vi "Dashboard Main.vi"() -> ()   [LabVIEW 2019]
uses:
  <vilib>/Utility/miscctls.llb/LVRowAndColumnTypeDef.ctl
  <vilib>/event_ctls.llb/eventvkey.ctl
  <vilib>/Rock Robotics/Network Tables/NT Read Numeric Array.vi
  <vilib>/Rock Robotics/Network Tables/NT Read Boolean.vi
  <vilib>/Rock Robotics/WPI/Dashboard/WPI_DashboardLogging Global.vi
panel:
  in  "Camera Settings Right":T1={"Frame Rate"=30, "Compression"=30, "Size"=1, "DB Camera Config"=FALSE} {"Frame Rate" scale=1.0..30.0; "Compression" scale=100.0..-1.0; "Size" items=["640x480", "320x240", "160x120"]}
  in  "Camera Name Right":string(combo)="No Camera Selection"
  out "Camera Perf":string
  in  "Camera Settings":T1={"Frame Rate"=30, "Compression"=30, "Size"=1, "DB Camera Config"=FALSE} {"Frame Rate" scale=1.0..30.0; "Compression" scale=100.0..-1.0; "Size" items=["640x480", "320x240", "160x120"]}
  in  "TCP":refnum<k5>
  in  "Rec Mode":enum32{"Stop", "Record", "Playback"}(radio)
  out "Robot IP":string
  out "Image Message":string="Timeout in Camera Communications"
  in  "Dashboard Tab":T2(tab)
  in  "Select Auto":string(combo)="Select Autonomous ..."
  out "NT Connection":bool
  out "MotorChart R":cluster{"Numeric":dbl, "Numeric":dbl}(graph)
  out "MotorChart L":cluster{"Numeric":dbl, "Numeric":dbl}(graph)
  out "MotorSliders R":cluster{"MotorSlide1":dbl, "MotorSlide2":dbl} {"MotorSlide2" scale=-1.0..1.0 scale format="%#_2e"; "MotorSlide1" scale=-1.0..1.0 scale format="%#_2e"}
  out "MotorSliders L":cluster{"MotorSlide1":dbl, "MotorSlide2":dbl} {"MotorSlide2" scale=-1.0..1.0 scale format="%#_2e"; "MotorSlide1" scale=-1.0..1.0 scale format="%#_2e"}
  out "Gyro":dbl(knob) scale=0.0..360.0
  out "JS1 Z":dbl(slide) scale=-1.0..1.0 scale format="%#_2e"
  out "JS1 Graph":cluster{"X":dbl, "Y":dbl}[](graph)
  out "JS1 Buttons":T3
  out "JS2 Z":dbl(slide) scale=-1.0..1.0 scale format="%#_2e"
  out "JS2 Graph":cluster{"X":dbl, "Y":dbl}[](graph)
  out "JS2 Buttons":T3
  out "Mode":T4(ring)=enum."Auto Disabled"
  out "Right Camera Perf":cluster{"Bandwidth (Mbps)":dbl, "FPS":dbl}
  out "Camera Image Right":T5(plugin-control)
  in  "DB/String 9":string
  in  "DB/String 8":string
  in  "DB/String 7":string
  in  "DB/String 6":string
  in  "DB/String 5":string
  in  "DB/String 4":string
  in  "DB/String 3":string
  in  "DB/String 2":string
  in  "DB/String 1":string
  in  "DB/String 0":string
  in  "DB/Slider 0":dbl(slide) scale=0.0..5.0
  in  "DB/Slider 1":dbl(slide) scale=0.0..5.0
  in  "DB/Slider 2":dbl(slide) scale=0.0..5.0
  in  "DB/Slider 3":dbl(slide) scale=0.0..5.0
  out "DB/LED 3":bool
  out "DB/LED 2":bool
  out "DB/LED 1":bool
  out "DB/LED 0":bool
  in  "DB/Button 3":bool
  in  "DB/Button 2":bool
  in  "DB/Button 1":bool
  in  "DB/Button 0":bool caption="New Name"
  out "Locked On":bool
  out "Current Shot":string
  out "Has Goal Target":bool
  out "Extendo Locked":bool
  out "Collector Position":string
  out "Ball Count":i32(slide) scale=0.0..5.0
  out "Spinny Thingy Color":string
  in  "Autonomous Mode":string(combo)
  in  "Test Slider":dbl(slide) scale=0.0..100.0 scale format="%#_3g"
  in  "On/Off":bool caption="Solenoid"
  in  "Test Name":u16(ring) items=["Select the test to run..."]
  in  "Test Tree":string(tree)
  in  "Motor":cluster{"Value":dbl, "Enable":bool} {"Value" scale=-1.0..1.0 scale format="%#_3g"}
  out "Progress":T6 {"Test Progress" scale=0.0..100.0}
  in  "Rev/Fwd":cluster{"Forward":bool, "Reverse":bool}
  in  "Test Ring":u16(ring) items=["Monochrome", "Color"]
  out "Cmd Status":string
  in  "Execute Command":bool
  in  "Command Params":string[][](table)
  in  "Command Selection":i32(listbox)
  in  "CheckList":i32(listbox)
  out "Tree":string(tree)
  out "Camera Image":T5(plugin-control)
  out "Background":bool
  in  "Camera Name":string(combo)="No Camera Selection"
  # "HW"
  # "HW"
  # "Joysticks"
  # "Drive Motors"
  # "Front"
  # "Right"
  # "Left"
  # "Back"
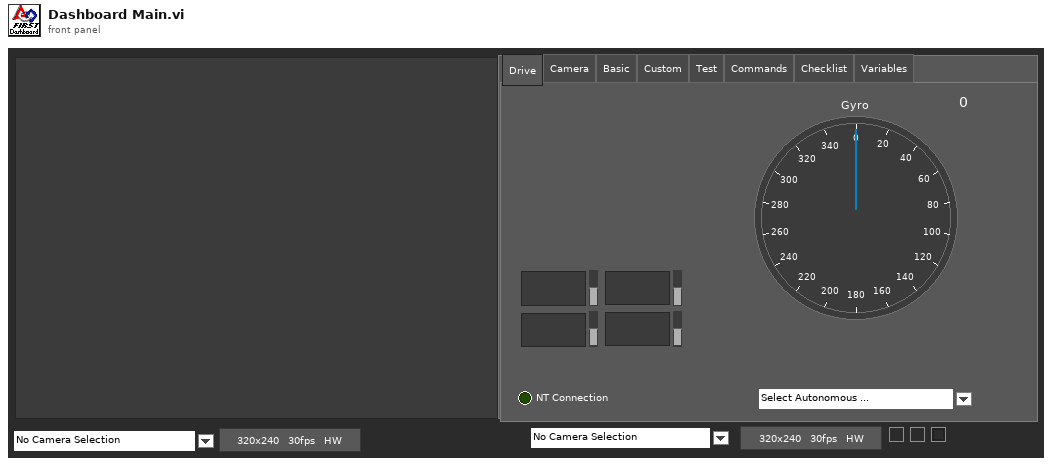
[diagram p1: front panel]
types:
  T1 = cluster{"Frame Rate":i32, "Compression":i32, "Size":u16, "DB Camera Config":bool}
  T2 = enum32{"Drive", "Camera", "Basic", "Custom", "Test", "Commands", "Checklist", "Variables"}
  T3 = cluster{bool, bool, bool, bool, bool, bool, bool, bool, bool, bool, bool, bool}
  T4 = enum8{"Tele-Op Disabled", "Tele-Op Enabled", "Auto Disabled", "Auto Enabled", "Test Disabled", "Test Enabled", "Disconnected", "No Code", "E-Stop"}
  T5 = typedef "IMAQ Image.ctl" = refnum<image>
  T6 = cluster{"Test Progress":u8, "Test Progress Text":string}
  T7 = cluster{"Save Path":path, "Interval (s)":dbl, "Keep":i32}
  T8 = typedef "Image Type" = u32
  T9 = cluster{"IDs":cluster{"RPC field ID":u16, "Unique ID":u16}, "String":string}
  T10 = cluster{"Error Strings":string, "Disable Counts":cluster{u16, u16}, "Rail Faults":cluster{u16, u16, u16}, "Robot IP":string, "DB Mode":u8, "Event Info":cluster{"Name":string, "Type":u8, "Number":u16, "Replay":u8}}
  T11 = cluster{"Storage":cluster{"Disk Free":u64, "RAM Block":u32, "RAM free":u32}, "CPU Utilization":cluster{"CPU % ISR":sgl, "CPU % Time Crit":sgl, "CPU % Timed Str":sgl, "CPU % High":sgl, "CPU % Above":sgl, "CPU % Normal":sgl, "CPU % Low":sgl}, "CAN":cluster{"% Bus Utilization":sgl, "Bus Off Cnt":u32, "TX_FIFO Full Cnt":u32, "Receive Error Cnt":u8, "Transmit Error Cnt":u8}, "HID":cluster{"HID Outputs":u32, "Rumble Low":u16, "Rumble High":u16}[]}
  T12 = cluster{"Status bits":cluster{"Test Mode":bool, "Autonomous":bool, "Enabled":bool, "Code Start":bool, "Brownout":bool, "Reserved 2":bool, "Reserved 3":bool, "E-Stop":bool}, "Code Trace":cluster{"Disabled":bool, "TeleOp":bool, "Auto":bool, "Test":bool}, "Controller Type":enum16{"unknown", "cRIO", "roboRio"}, "Code?":enum16{"unknown", "noCode", "code"}, "Battery V":dbl}
  T13 = cluster{"Control Bits":cluster{"TestMode":bool, "Autonomous":bool, "Enabled":bool, "FMS Present":bool, bool, bool, bool, "E-Stop":bool}, "Team Station ":u8, "Countdown":sgl, "Joystick Values":cluster{"Axes":dbl[], "Buttons":bool[], "POVs":i16[]}[]}
  T14 = cluster{"Axes":dbl[], "Buttons":bool[], "POVs":i16[]}[]
  T15 = cluster{"Axes":dbl[], "Buttons":bool[], "POVs":i16[]}
  T16 = cluster{"Buttons[0]":bool, "Buttons[1]":bool, "Buttons[2]":bool, "Buttons[3]":bool, "Buttons[4]":bool, "Buttons[5]":bool, "Buttons[6]":bool, "Buttons[7]":bool, "Buttons[8]":bool, "Buttons[9]":bool, "Buttons[10]":bool, "Buttons[11]":bool}
  T17 = cluster{"Camera Image":refnum<vi>, "Dashboard Tab":refnum<vi>, "Background":refnum<vi>, "Rec Mode":refnum<vi>, "Test Slider":refnum<vi>, "On/Off ":refnum<vi>, "Test Ring":refnum<vi>, "Rev/Fwd":refnum<vi>, "Test Name":refnum<vi>, "Motor":refnum<vi>, "Progress":refnum<vi>, "CheckList":refnum<vi>, "Tree":refnum<vi>, "Test Tree":refnum<vi>, "Command Params":refnum<vi>, "Command Selection":refnum<vi>, "Execute Command":refnum<vi>, "Cmd Status":refnum<vi>, "Camera Settings":refnum<vi>, "Camera Name":refnum<vi>, "Camera Perf":refnum<vi>, "Camera Settings Right":refnum<vi>, "Camera Name Right":refnum<vi>, "Camera Image Right":refnum<vi>}
  T18 = cluster{"Global Rectangle":i32[], "Contours":cluster{"Contour Type":u32, "ROI Type":u32, "Points":i32[]}[]}
  T19 = cluster{"Camera Name":string, string, "Saved DB Images Info":cluster{"Save Path":path, "Interval (s)":dbl, "Keep":i32}}
  T20 = cluster{"Camera Name Right":string, string, "Saved DB Images Info":cluster{"Save Path":path, "Interval (s)":dbl, "Keep":i32}}
  T21 = cluster{"Operation":enum16{"Update", "Clear"}, "Color Box":u32}[]
  T22 = typedef "eventvkey.ctl" = enum16{"ASCII", "Enter", "Return", "Shift", "Ctrl", "Alt", "Cmd", "Opt", "Caps", "NumLock", "Clear", "Break", "Up", "Down", "Left", "Right", "Insert", "Delete", "Home", "End", "PageUp", "PageDown", "Escape", "Help", "Pause", "ScrollLock", "F1", "F2", "F3", "F4", "F5", "F6", "F7", "F8", "F9", "F10", "F11", "F12", "F13", "F14", "F15", "F16", "F17", "F18", "F19", "F20", "F21", "F22", "F23", "F24", "Play", "VolumeUp", "VolumeDown", "Mute", "Two Byte Char"}
  T23 = cluster{"Image Size":bool, "Image Type":bool, "Pixel Value":bool, "ROI Information":bool, "Zoom Factor":bool}
  T24 = cluster{"Operation":enum16{"Update", "Clear"}, "Color Box":u32}
  T25 = typedef "LVRowAndColumnTypeDef.ctl" = cluster{"Row":i32, "Column":i32}
  T26 = cluster{"Shift":bool, "Ctrl":bool, "Alt":bool, "Cmd":bool, "Opt":bool}
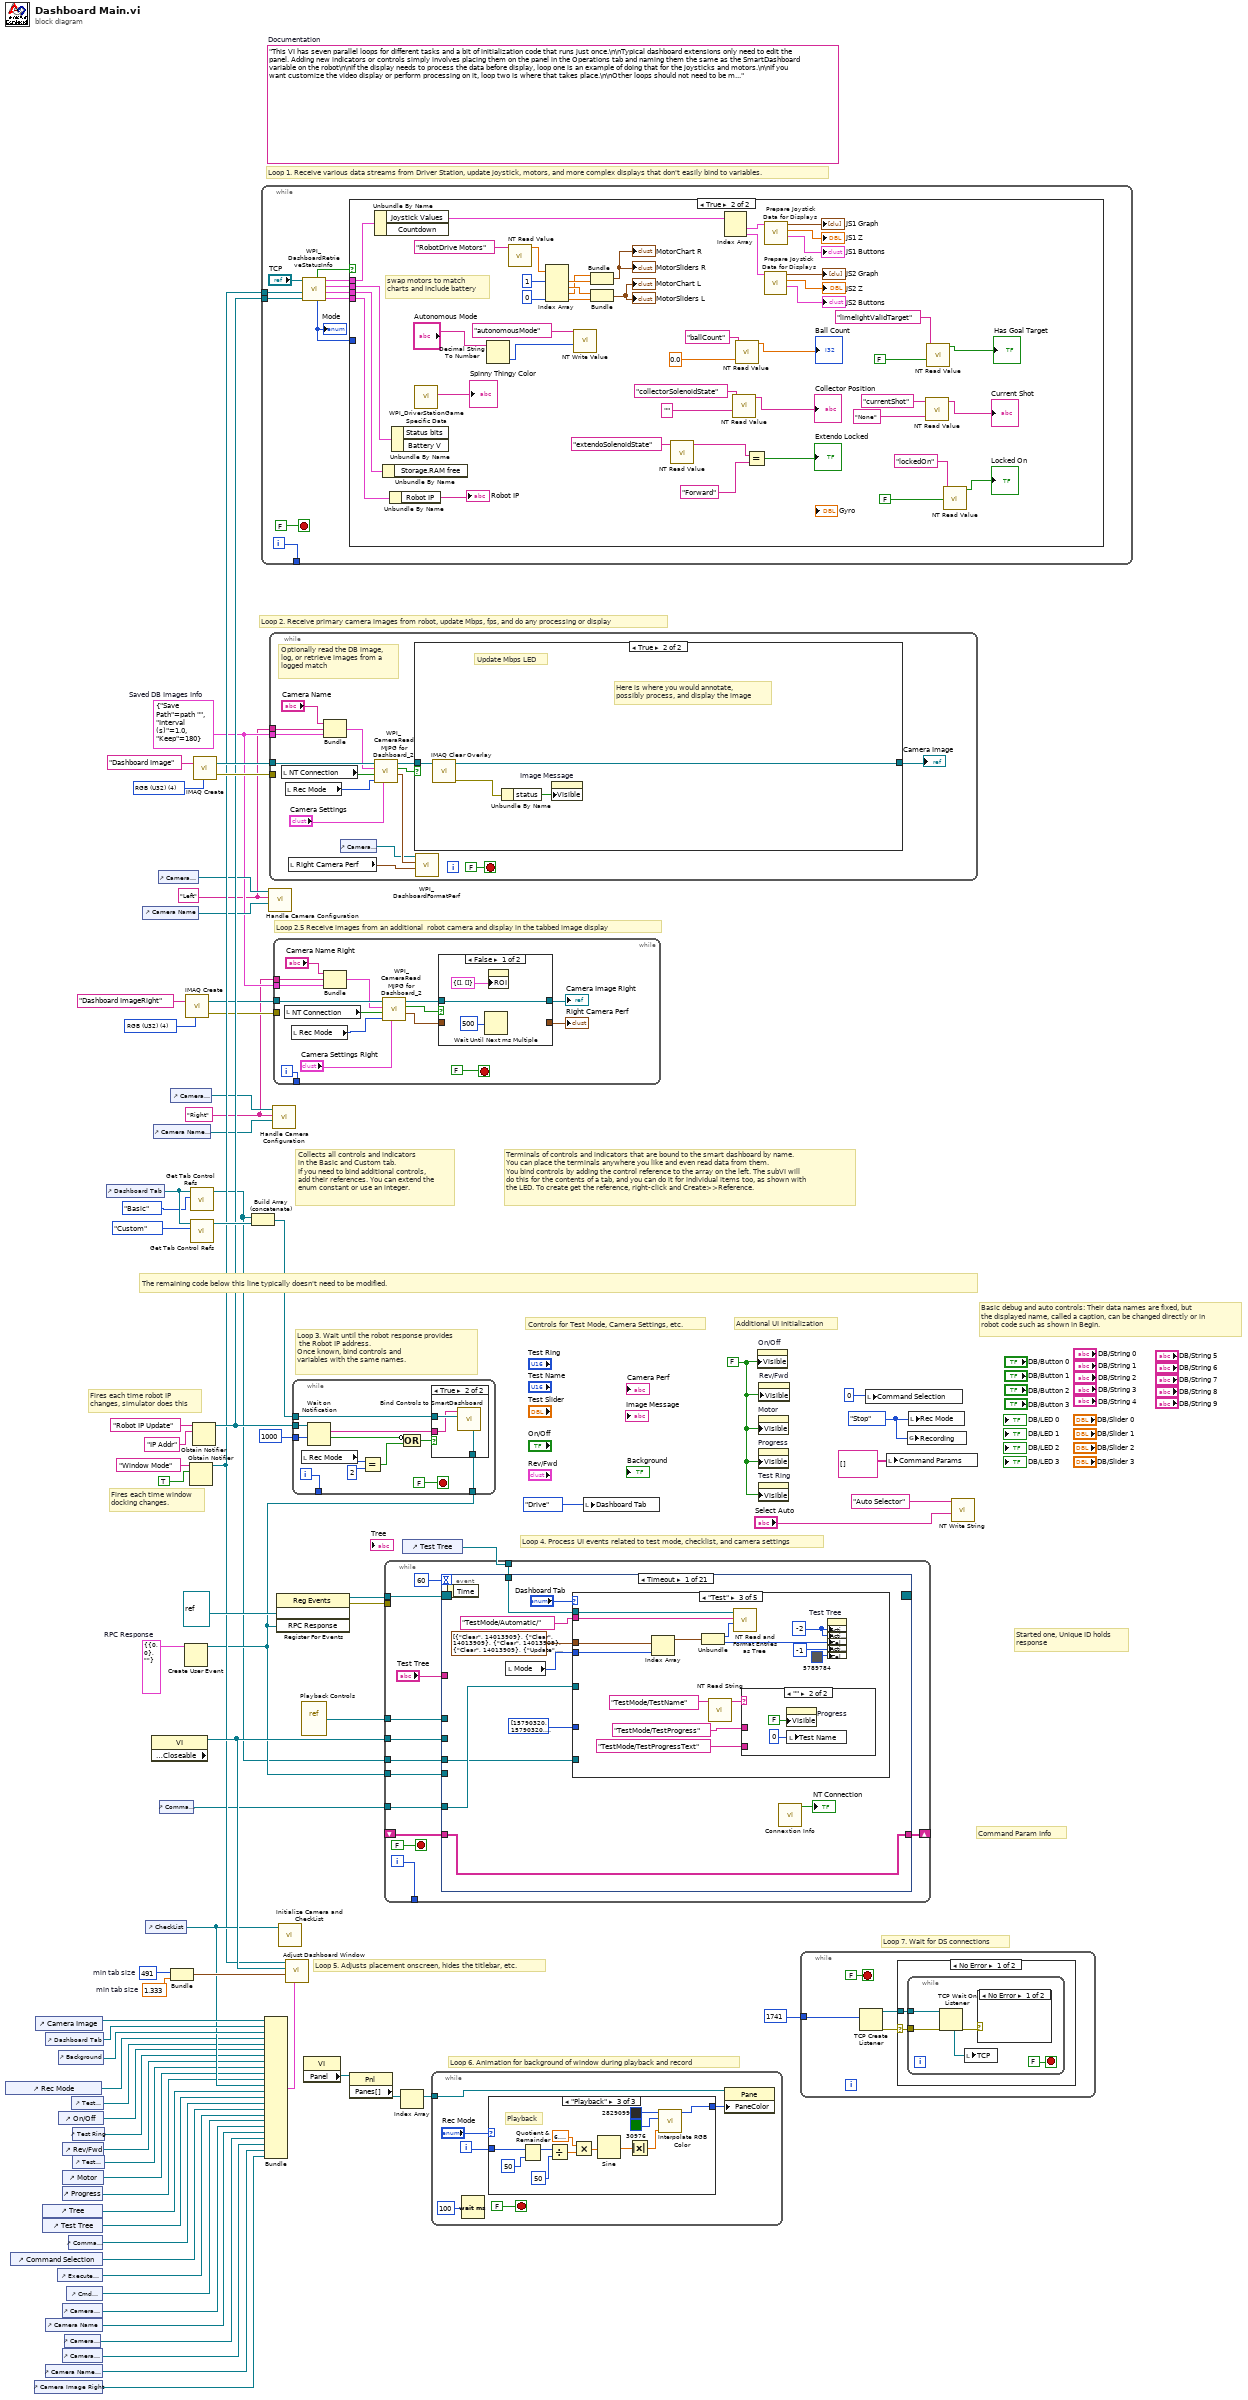
[diagram p0: block diagram]
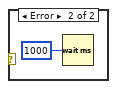
[diagram p3: hidden frame]
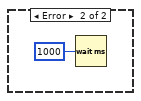
[diagram p4: hidden frame]
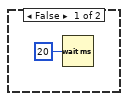
[diagram p5: hidden frame]
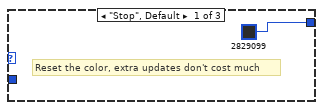
[diagram p6: hidden frame]
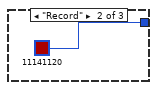
[diagram p7: hidden frame]
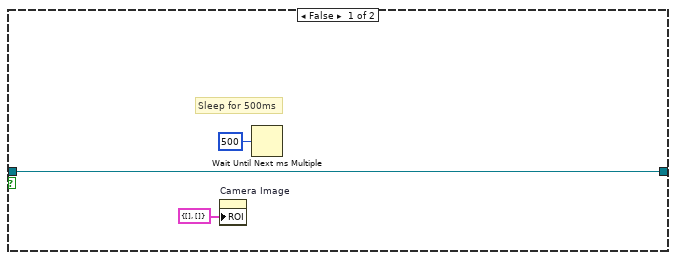
[diagram p9: hidden frame]
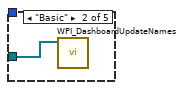
[diagram p11: hidden frame]
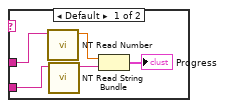
[diagram p12: hidden frame]
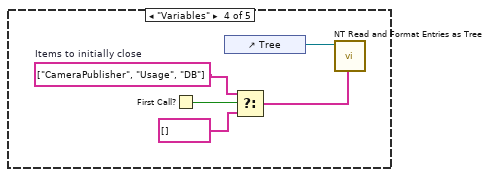
[diagram p13: hidden frame]
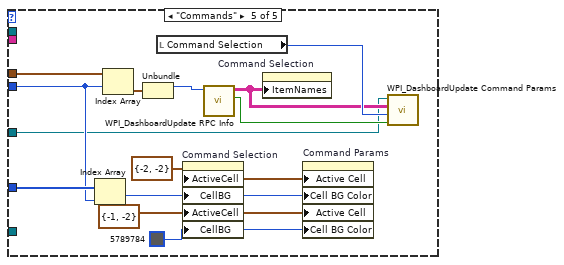
[diagram p14: hidden frame]
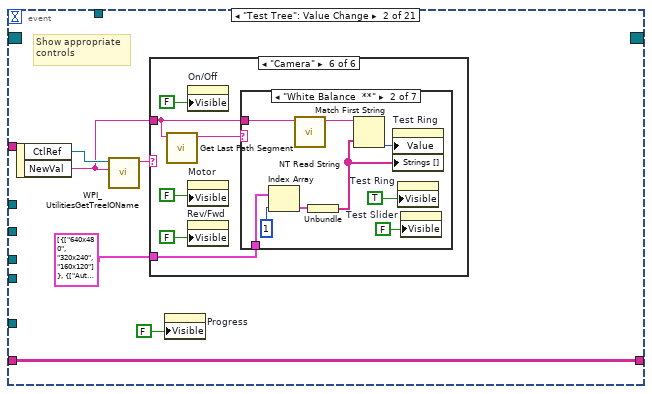
[diagram p15: hidden frame]
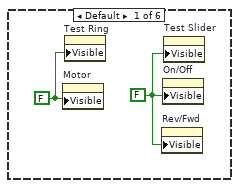
[diagram p16: hidden frame]
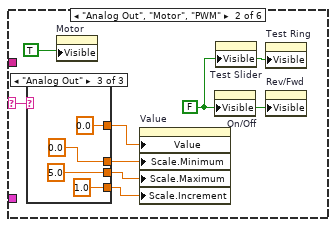
[diagram p17: hidden frame]
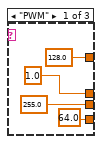
[diagram p18: hidden frame]
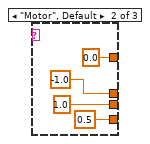
[diagram p19: hidden frame]
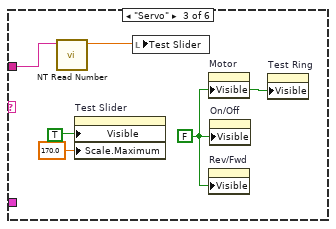
[diagram p20: hidden frame]
diagram:
  w3 = T7 {"Save Path"=path "", "Interval (s)"=1.0, "Keep"=180}  # Saved DB Images Info
  w2 = "Right"
  w1 = "Left"
  w13 = T8 4 items=["Grayscale (U8)", "Grayscale (I16)", "Grayscale (SGL)", "Complex (CSG)", "RGB (U32)", "HSL (U32)", "RGB (U64)"] ("Image Type")
  w29 = T9 {"IDs"={"RPC field ID"=0, "Unique ID"=0}, "String"=""}  # RPC Response
  w52 = 491  # min tab size
  w51 = 1.333  # min tab size
  w59 = enum32{"Stop", "Record", "Playback"}."Stop" ("Rec Mode")
  w36 = FALSE ("Visible")
  (unwired) "This VI has seven parallel loops for different tasks and a bit of initialization code that runs just once.\n\nTypical dashboard extensions only need to edit the panel. Adding new indicators or controls simply involves placing them on the panel in the Operations tab and naming them the same as the SmartDashboard variable on the robot\n\nIf the display needs to process the data before display, loop one is an example of doing that for the joysticks and motors.\n\nIf you want customize the video display or perform processing on it, loop two is where that takes place.\n\nOther loops should not need to be modified. They are pretty standard, and document the task they perform."  # Documentation
  w76 = T8 4 items=["Grayscale (U8)", "Grayscale (I16)", "Grayscale (SGL)", "Complex (CSG)", "RGB (U32)", "HSL (U32)", "RGB (U64)"] ("Image Type")
  # "Loop 2.5 Receive images from an additional  robot camera and display in the tabbed image display"
  # "Command Param Info"
  # "Started one, Unique ID holds\nresponse"
  # "Loop 7. Wait for DS connections"
  # "Basic debug and auto controls: Their data names are fixed, but\nthe displayed name, called a caption, can be changed directly or in\nrobot code such as shown in Begin."
  # "Controls for Test Mode, Camera Settings, etc."
  # "Additional UI Initialization"
  # "Loop 6. Animation for background of window during playback and record"
  # "Fires each time robot IP\nchanges, simulator does this"
  # "Fires each time window\ndocking changes."
  # "Collects all controls and indicators\nin the Basic and Custom tab.\nIf you need to bind additional controls,\nadd their references. You can extend the\nenum constant or use an integer."
  # "The remaining code below this line typically doesn't need to be modified."
  # "Loop 4. Process UI events related to test mode, checklist, and camera settings"
  # "Terminals of controls and indicators that are bound to the smart dashboard by name.\nYou can place the terminals anywhere you like and even read data from them.\nYou bind controls by adding the control reference to the array on the left. The subVI will\ndo this for the contents of a tab, and you can do it for individual items too, as shown with\nthe LED. To create get the reference, right-click and Create>>Reference."
  # "Loop 3. Wait until the robot response provides\n the Robot IP address.\nOnce known, bind controls and\nvariables with the same names."
  # "Loop 5. Adjusts placement onscreen, hides the titlebar, etc."
  # "Loop 1. Receive various data streams from Driver Station, update joystick, motors, and more complex displays that don't easily bind to variables."
  # "Loop 2. Receive primary camera images from robot, update Mbps, fps, and do any processing or display"
  n1 = control-ref of="Rec Mode"() -> (w42:refnum<vi>)
  n2 = control-ref of="Command Selection"() -> (w28:refnum<vi>)
  n3 = control-ref of="Camera Image Right"() -> (w6:refnum<vi>)
  n4 = control-ref of="Camera Image"() -> (w54:refnum<vi>)
  n5 = control-ref of="Tree"() -> (w46:refnum<vi>)
  n6 = control-ref of="Test Tree"() -> (w45:refnum<vi>)
  n7 = control-ref of="Dashboard Tab"() -> (w53:refnum<vi>)
  n8 = control-ref of="Camera Name"() -> (w19:refnum<vi>)
  n9 = control-ref of="Camera Name Right"() -> (w7:refnum<vi>)
  n10 = control-ref of="Execute Command"() -> (w30:refnum<vi>)
  n11 = control-ref of="Background"() -> (w49:refnum<vi>)
  n12 = control-ref of="On/Off"() -> (w40:refnum<vi>)
  n13 = control-ref of="Progress"() -> (w37:refnum<vi>)
  n14 = control-ref of="Camera Settings"() -> (w20:refnum<vi>)
  n15 = control-ref of="Camera Settings Right"() -> (w8:refnum<vi>)
  n16 = control-ref of="Rev/Fwd"() -> (w38:refnum<vi>)
  n17 = control-ref of="Motor"() -> (w43:refnum<vi>)
  n18 = control-ref of="Camera Perf"() -> (w18:refnum<vi>)
  n19 = control-ref of="Cmd Status"() -> (w24:refnum<vi>)
  n20 = control-ref of="Command Params"() -> (w31:refnum<vi>)
  n21 = control-ref of="Test Slider"() -> (w41:refnum<vi>)
  n22 = control-ref of="Test Ring"() -> (w39:refnum<vi>)
  n23 = control-ref of="Test Name"() -> (w44:refnum<vi>)
  n24 = control-ref of="Dashboard Tab"() -> (w57:refnum<vi>)
  n25 = control-ref of="Camera Name"() -> (w21:refnum<vi>)
  n26 = control-ref of="CheckList"() -> (w47:refnum<vi>)
  n27 = property class="VI" props=["Front Panel.Closeable"]() -> (reference out=w58:refnum<vi>)  [unwired: 2 in, 2 out]
  n28 = control-ref of="Camera Name Right"() -> (w9:refnum<vi>)
  n29 = control-ref of="Camera Settings"() -> (w22:refnum<vi>)
  n30 = control-ref of="Command Params"() -> (w23:refnum<vi>)
  n31 = control-ref of="Camera Settings Right"() -> (w10:refnum<vi>)
  n32 = Bundle("min tab size"=w52, "min tab size"=w51) -> (w50:cluster{"min tab size":i32, "min tab size":dbl})  [unwired: 1 in]
  n33 = Create User Event(user event datatype=w29) -> (user event=w25:refnum<user-event>)  [unwired: 1 in, 1 out]
  n34 = call "IMAQ Create"("Image Name"="Dashboard ImageRight", "Image Type"=w13) -> ("New Image"=w12:T5, "error out"=w11:errorcluster)  [unwired: 2 in, 1 out]
  n35 = Obtain Notifier(name (unnamed)="Window Mode", notification data type=TRUE) -> (notifier out=w34:refnum<notifier>)  [unwired: 2 in, 2 out]
  n36 = call <vilib>:"Get Tab Control Refs.vi"("Page Index"=T2."Basic" ("Dashboard Tab"), "TabControl in"=w57) -> ("ControlsOnPage"=w17:refnum<vi>[])  [unwired: 9 in]
  n37 = call <vilib>:"Get Tab Control Refs.vi"("Page Index"=T2."Custom" ("Dashboard Tab"), "TabControl in"=w57) -> ("ControlsOnPage"=w56:refnum<vi>[])  [unwired: 9 in]
  n38 = Obtain Notifier(name (unnamed)="Robot IP Update", notification data type="IP Addr" ("name (unnamed)")) -> (notifier out=w35:refnum<notifier>)  [unwired: 2 in, 2 out]
  n39 = call "IMAQ Create"("Image Name"="Dashboard Image", "Image Type"=w76) -> ("New Image"=w74:T5, "error out"=w73:errorcluster)  [unwired: 2 in, 1 out]
  n40 = Build Array (concatenate)(w17, w56) -> (w55:refnum<vi>[])
  n41 = while {
    tunnel: [w86] -> _
    tunnel: w35 -> [w80]
    tunnel: w34 -> [w77]
    i -> [w86]
    stop <- FALSE stop-if-true
    n42 = call <vilib>:"WPI_DashboardRetrieveStatusInfo.vi"("Binding Refnum"=w80, "Window Mode Notifier"=w77, "TCP Cnx"="TCP") -> ("Power and Errors"=w81:T10, "Robot Metrics"=w84:T11, "Status Info"=w85:T12, "Control Info"=w82:T13, "Robot Mode"=w79:T4, "Process?"=w83:bool)  [unwired: 3 in]
    "Mode" <- w79
    n43 = case shown="True" w83 {
      tunnel: w85 -> [_ w135]
      tunnel: w84 -> [_ w134]
      tunnel: w82 -> [_ w133]
      tunnel: w81 -> [_ w132]
      tunnel: w79 -> [_ _]
      frame False {
        n44 = Wait (ms)(milliseconds to wait=u32 20) -> ()  [unwired: 1 out]
      }
      frame True {
        # "swap motors to match\ncharts and include battery"
        n45 = Unbundle By Name(w133) -> ("Joystick Values"=w123:T14)  [unwired: 1 out]
        n46 = Unbundle By Name(w134) -> ()  [unwired: 1 out]
        n47 = Unbundle By Name(w132) -> ("Robot IP"=→"Robot IP":string)
        n48 = Unbundle By Name(w135) -> ()  [unwired: 2 out]
        n49 = call <vilib>:"WPI_DriverStationGame Specific Data.vi"() -> ("Game Specific Data"=→"Spinny Thingy Color":string)  [unwired: 11 in]
        n50 = Decimal String To Number(string="Autonomous Mode") -> (number=w110:i32)  [unwired: 2 in, 1 out]
        n51 = call-poly <vilib>:"NT Read Value.vi"("Name"="RobotDrive Motors") -> ("Numeric Array"=w113:dbl[])  [unwired: 9 in, 1 out]
        n52 = Index Array(array=w113, index #1=1, index #4=0) -> (element #1=w127:dbl, element #2=w128:dbl, element #3=w126:dbl, element #4=w131:dbl)  [unwired: 2 in]
        n53 = call-poly <vilib>:"NT Write Value.vi"("Numeric"=w110, "Name"="autonomousMode") -> ()  [unwired: 9 in, 1 out]
        n54 = Bundle("Numeric"=w126, "Numeric"=w127) -> (→"MotorChart R" →"MotorSliders R":cluster{"Numeric":dbl, "Numeric":dbl})  [unwired: 1 in]
        n55 = Bundle("Numeric"=w128, "Numeric"=w131) -> (→"MotorChart L" →"MotorSliders L":cluster{"Numeric":dbl, "Numeric":dbl})  [unwired: 1 in]
        n56 = call-poly <vilib>:"NT Read Value.vi"("Name"="extendoSolenoidState") -> ("String"=w100:string)  [unwired: 9 in, 1 out]
        n57 = Index Array(array=w123) -> (element #1=w122:T15, element #2=w118:T15)  [unwired: 2 in]
        n58 = call-poly <vilib>:"NT Read Value.vi"("Default Value"="", "Name"="collectorSolenoidState") -> ("String"=→"Collector Position":string)  [unwired: 8 in, 1 out]
        n59 = call-poly <vilib>:"NT Read Value.vi"("Default Value"=0.0, "Name"="ballCount") -> ("Numeric"=→"Ball Count":dbl)  [unwired: 8 in, 1 out]
        n60 = Equal?(x=w100, y="Forward") -> (x = y?=→"Extendo Locked":bool)
        n61 = call "Prepare Joystick Data for Displays.vi"("Joystick Values"=w118) -> ("Buttons"=→"JS2 Buttons":T16, "Z Axis"=→"JS2 Z":dbl, "Cartesian Data"=→"JS2 Graph":cluster{"X axis":dbl, "X axis":dbl}[])  [unwired: 8 in]
        n62 = call "Prepare Joystick Data for Displays.vi"("Joystick Values"=w122) -> ("Buttons"=→"JS1 Buttons":T16, "Z Axis"=→"JS1 Z":dbl, "Cartesian Data"=→"JS1 Graph":cluster{"X axis":dbl, "X axis":dbl}[])  [unwired: 8 in]
        n63 = call-poly <vilib>:"NT Read Value.vi"("Default Value"="None", "Name"="currentShot") -> ("String"=→"Current Shot":string)  [unwired: 8 in, 1 out]
        n64 = call-poly <vilib>:"NT Read Value.vi"("Default Value"=FALSE, "Name"="limelightValidTarget") -> ("Boolean"=→"Has Goal Target":bool)  [unwired: 8 in, 1 out]
        n65 = call-poly <vilib>:"NT Read Value.vi"("Default Value"=FALSE, "Name"="lockedOn") -> ("Boolean"=→"Locked On":bool)  [unwired: 8 in, 1 out]
      }
    }
  }
  n66 = Bundle("Camera Image"=w54, "Dashboard Tab"=w53, "Background"=w49, "Rec Mode"=w42, "Test Slider"=w41, "On/Off"=w40, "Test Ring"=w39, "Rev/Fwd"=w38, "Test Name"=w44, "Motor"=w43, "Progress"=w37, "CheckList"=w47, "Tree"=w46, "Test Tree"=w45, "Command Params"=w31, "Command Selection"=w28, "Execute Command"=w30, "Cmd Status"=w24, "Camera Settings"=w20, "Camera Name"=w19, "Camera Perf"=w18, "Camera Settings Right"=w8, "Camera Name Right"=w7, "Camera Image Right"=w6) -> (w48:T17)  [unwired: 1 in]
  n67 = call "Handle Camera Configuration.vi"("CameraNameRef"=w21, "Display Name"=w1, "ClusterRef"=w22) -> ()  [unwired: 9 in]
  n68 = while {
    tunnel: w74 -> [w149]
    tunnel: w73 -> [_]
    tunnel: w3 -> [w142]
    tunnel: w1 -> [w139]
    stop <- FALSE stop-if-true
    # "Optionally read the DB image,\nlog, or retrieve images from a\nlogged match"
    n69 = local read "NT Connection"() -> (w143:bool)
    n70 = local read "Rec Mode"() -> (w146:enum32{"Stop", "Record", "Playback"})
    n71 = local read "Right Camera Perf"() -> (w137:cluster{"Bandwidth (Mbps)":dbl, "FPS":dbl})
    n72 = Bundle("Camera Name"="Camera Name", w139, "Saved DB Images Info"=w142) -> (w141:T19)  [unwired: 1 in]
    n73 = control-ref of="Camera Perf"() -> (w136:refnum<vi>)
    n74 = call <vilib>:"WPI_CameraRead MJPG for Dashboard_2.vi"("Camera Settings"="Camera Settings", "Rec Mode"=w146, "NT Connection"=w143, "Capture Info"=w141, "Image in"=w149) -> ("perf info"=w138:cluster{"Bandwidth (Mbps)":dbl, "fps":dbl}, "Active"=w147:bool, "Image\\ out"=w148:T5)  [unwired: 4 in]
    n75 = case shown="True" w147 {
      tunnel: w148 -> [w152 w155]
      tunnel: [w152 w154] -> w144
      frame False {
        # "Sleep for 500ms"
        n76 = property on="Camera Image" class="ImageControl"("ROI"=T18 {"Global Rectangle"=[], "Contours"=[]}) -> ()  [unwired: 2 in, 2 out]
        n77 = Wait Until Next ms Multiple(millisecond multiple=u32 500) -> ()  [unwired: 1 out]
      }
      frame True {
        # "Here is where you would annotate,\npossibly process, and display the image"
        # "Update Mbps LED"
        n78 = call "IMAQ Clear Overlay"("Image"=w155) -> ("error out"=w156:errorcluster, "Image Out"=w154:T5)  [unwired: 2 in, 7 out]
        n79 = Unbundle By Name(w156) -> ("status"=w157:bool)
        n80 = property on="Image Message" class="Str"("Visible"=w157) -> ()  [unwired: 2 in, 2 out]
      }
    }
    "Camera Image" <- w144
    n81 = call <vilib>:"WPI_DashboardFormatPerf.vi"("Right Camera Perf"=w137, "Performance"=w138, "String in"=w136) -> ()  [unwired: 9 in]
  }
  n82 = call "Handle Camera Configuration.vi"("CameraNameRef"=w9, "Display Name"=w2, "ClusterRef"=w10) -> ()  [unwired: 9 in]
  n83 = while {
    tunnel: w12 -> [w172]
    tunnel: w11 -> [_]
    tunnel: [w167] -> _
    tunnel: w3 -> [w163]
    tunnel: w2 -> [w160]
    i -> [w167]
    stop <- FALSE stop-if-true
    n84 = local read "NT Connection"() -> (w164:bool)
    n85 = local read "Rec Mode"() -> (w171:enum32{"Stop", "Record", "Playback"})
    n86 = Bundle("Camera Name Right"="Camera Name Right", w160, "Saved DB Images Info"=w163) -> (w162:T20)  [unwired: 1 in]
    n87 = call <vilib>:"WPI_CameraRead MJPG for Dashboard_2.vi"("Camera Settings"="Camera Settings Right", "Rec Mode"=w171, "NT Connection"=w164, "Capture Info"=w162, "Image in"=w172) -> ("perf info"=w158:cluster{"Bandwidth (Mbps)":dbl, "fps":dbl}, "Active"=w166:bool, "Image\\ out"=w169:T5)  [unwired: 4 in]
    n88 = case shown="False" w166 {
      tunnel: w169 -> [w174 w177]
      tunnel: [w174 w177] -> w165
      tunnel: [_ w176] -> w159
      tunnel: w158 -> [_ w176]
      frame False {
        n89 = Wait Until Next ms Multiple(millisecond multiple=u32 500) -> ()  [unwired: 1 out]
        n90 = property on="Camera Image Right" class="ImageControl"("ROI"=T18 {"Global Rectangle"=[], "Contours"=[]}) -> ()  [unwired: 2 in, 2 out]
      }
      frame True {
      }
    }
    "Camera Image Right" <- w165
    "Right Camera Perf" <- w159
  }
  n91 = register-events(refnum<vi> refnum, w25) -> (reference out=w63:refnum<event-registration>, error out=w62:errorcluster)  [unwired: 2 in]
  n92 = call "Initialize Camera and CheckList.vi"("ListBox in"=w47) -> ()  [unwired: 11 in]
  n93 = call "Adjust Dashboard Window.vi"("Sizing Refnums"=w48, "Size Constraints"=w50, "VI"=w58, "WIn Mode"=w34) -> ()  [unwired: 8 in]
  n94 = while {
    tunnel: w55 -> [w189]
    tunnel: w35 -> [w187]
    tunnel: [w185] -> _
    tunnel: u32 1000 ("milliseconds to wait") -> [w184]
    tunnel: w25 -> [w178]
    i -> [w185]
    stop <- FALSE stop-if-true
    n95 = local read "Rec Mode"() -> (w180:enum32{"Stop", "Record", "Playback"})
    n96 = Wait on Notification(notifier=w187, timeout in ms (-1)=w184) -> (notification=w186:string, timed out?=w182:bool)  [unwired: 2 in, 2 out]
    n97 = Equal?(x=w180, y=u16 2 ("Rec Mode")) -> (x = y?=w181:bool)
    n98 = Compound Arithmetic op=OR(invert w182, w181) -> (w183:bool)
    n99 = case shown="True" w183 {
      tunnel: w189 -> [_ w192]
      tunnel: w186 -> [_ w191]
      tunnel: w178 -> [_ w190]
      frame False {
      }
      frame True {
        n100 = call <vilib>:"Bind Controls to SmartDashboard.vi"("RPC ref"=w190, "Bound Control Refs"=w192, "Server IP Address"=w191) -> ()  [unwired: 9 in]
      }
    }
  }
  n101 = vi-ref "Playback Controls.vi"() -> (w64:refnum<vi>)
  n102 = property class="VI"() -> ("Panel"=w66:refnum<vi>)  [unwired: 2 in, 2 out]
  n103 = property class="Pnl"(reference=w66) -> ("Panes[]"=w67:refnum<vi>[])  [unwired: 1 in, 2 out]
  n104 = Index Array(array=w67) -> (element=w65:refnum<vi>)  [unwired: 1 in]
  n105 = control-ref of="Test Tree"() -> (w68:refnum<vi>)
  n106 = while {
    tunnel: [w202] -> _
    tunnel: w68 -> [w201]
    tunnel: w64 -> [w200]
    tunnel: w63 -> [w199]
    tunnel: w62 -> [_]
    tunnel: w58 -> [w198]
    tunnel: w25 -> [w197]
    tunnel: w23 -> [w196]
    shift-right: [w195] -> _
    shift-left: _ -> [w194]
    tunnel: w17 -> [w193]
    i -> [w202]
    stop <- FALSE stop-if-true
    n107 = event shown="[0] Timeout" {
      selector: w199 -> [_ _ _ _ _ _ _ _ _ _ _ _ _ _ _ _ _ _ _ _ _]
      dyn-events: [_ _ _ _ _ _ _ _ _ _ _ _ _ _ _ _ w462 _ _ _ _] -> _
      timeout: u32 60 ("milliseconds to wait") -> [_ _ _ _ _ _ _ _ _ _ _ _ _ _ _ _ _ _ _ _ _]
      tunnel: w201 -> [w214 _ _ _ _ _ _ _ _ _ _ _ _ _ _ _ _ _ _ _ _]
      tunnel: "Test Tree" -> [_ _ _ _ _ _ _ _ _ _ _ w429 w437 w439 w443 w451 _ _ _ _ _]
      tunnel: w200 -> [_ _ _ _ _ _ _ _ _ _ _ _ _ _ _ _ w464 _ w482 _ _]
      tunnel: w198 -> [_ _ _ _ _ _ _ _ _ _ _ _ _ _ _ _ w460 _ _ _ _]
      tunnel: w197 -> [_ _ _ _ _ _ _ _ _ _ _ _ _ _ _ _ w458 _ _ _ _]
      tunnel: w196 -> [w209 _ _ _ _ _ w380 _ _ _ _ _ _ _ _ _ _ _ _ _ _]
      tunnel: [w208 w257 w359 w364 w373 w377 w378 w387 w397 w404 w416 w428 w435 w438 w442 w450 w457 w477 w479 w483 w496] -> w195
      tunnel: w194 -> [w208 w257 w359 w364 w373 w377 w378 _ _ w404 w416 w428 w435 w438 w442 w450 w457 w477 w479 w483 w496]
      tunnel: w193 -> [w206 _ _ _ _ _ _ _ _ _ _ _ _ _ _ _ _ _ _ _ _]
      event Timeout {
        n108 = event-data() -> ()  [unwired: 1 in, 1 out]
        n109 = local read "Mode"() -> (w211:T4)
        n110 = case shown="\"Test\"" "Dashboard Tab" {
          tunnel: w214 -> [_ _ w230 _ _]
          tunnel: "TestMode/Automatic/" ("Name Pattern") -> [_ _ w229 _ _]
          tunnel: T21 [{"Operation"=enum."Clear", "Color Box"=14013909}, {"Operation"=enum."Clear", "Color Box"=14013909}, {"Operation"=enum."Clear", "Color Box"=14013909}, {"Operation"=enum."Clear", "Color Box"=14013909}, {"Operation"=enum."Update", "Color Box"=14013909}, {"Operation"=enum."Update", "Color Box"=16777215}, {"Operation"=enum."Clear", "Color Box"=14013909}, {"Operation"=enum."Clear", "Color Box"=14013909}, {"Operation"=enum."Clear", "Color Box"=14013909}] -> [_ _ w222 _ w250]
          tunnel: w211 -> [_ _ w221 _ w249]
          tunnel: u32[] [15790320, 15790320, 15790320, 15790320, 16777215, 16777215, 15790320, 15790320, 15790320] -> [_ _ _ _ w255]
          tunnel: w209 -> [_ _ _ _ w243]
          tunnel: w206 -> [_ w216 _ _ _]
          frame "Custom", Default {
          }
          frame "Basic" {
            n111 = call <vilib>:"WPI_DashboardUpdateNames.vi"("Controls on Tab"=w216) -> ()  [unwired: 11 in]
          }
          frame "Test" {
            w228 = -2 ("Active Item:Row Number")
            n112 = Index Array(array=w222, index=w221) -> (element=w223:T24)
            n113 = Unbundle(w223) -> ("Operation"=w224:enum16{"Update", "Clear"}, "Color Box"=w225:u32)
            n114 = call <vilib>:"NT Read String.vi"("Name"="TestMode/TestName") -> ("String"=w219:string)  [unwired: 9 in, 1 out]
            n115 = call <vilib>:"NT Read and Format Entries as Tree.vi"("Operation"=w224, "Name Pattern"=w229, "Tree Refnum"=w230) -> ()  [unwired: 7 in, 2 out]
            n116 = case shown="\"\"" w219 {
              tunnel: "TestMode/TestProgress" ("Name") -> [w232 _]
              tunnel: "TestMode/TestProgressText" ("Name") -> [w231 _]
              frame Default {
                n117 = call <vilib>:"NT Read Number.vi"("Name"=w232) -> ("Numeric"=w233:dbl)  [unwired: 9 in, 1 out]
                n118 = call <vilib>:"NT Read String.vi"("Name"=w231) -> ("String"=w234:string)  [unwired: 9 in, 1 out]
                n119 = Bundle("Numeric"=w233, "String"=w234) -> (→"Progress":cluster{"Numeric":dbl, "String":string})  [unwired: 1 in]
              }
              frame "" {
                n120 = property on="Progress" class="Clust (strict)"("Visible"=FALSE) -> ()  [unwired: 2 in, 2 out]
                n121 = local write "Test Name"(u16 0) -> ()
              }
            }
            n122 = property on="Test Tree" class="Tree (strict)"("Active Item Row Number"=w228, "ActiveColNum"=w228, "CellBG"=w225, "Active Item Row Number"=-1 ("Active Item:Row Number"), "CellBG"=u32 5789784 ("Color Box")) -> ()  [unwired: 2 in, 2 out]
          }
          frame "Variables" {
            w240 = string[] ["CameraPublisher", "Usage", "DB"]  # Items to initially close
            n123 = First Call?() -> (First Call?: T/F=w241:bool)
            n124 = control-ref of="Tree"() -> (w242:refnum<vi>)
            n125 = Select(t=w240, s=w241, f=string[] []) -> (s? t:f=w238:string[])
            n126 = call <vilib>:"NT Read and Format Entries as Tree.vi"("Tags to  Close"=w238, "Tree Refnum"=w242) -> ()  [unwired: 8 in, 2 out]
          }
          frame "Commands" {
            w251 = u32 5789784 ("Color Box")
            w252 = T25 {"Row"=-1, "Column"=-2} ("Active Cell:Active Cell")
            w254 = T25 {"Row"=-2, "Column"=-2} ("Active Cell:Active Cell")
            n127 = Index Array(array=w255, index=w249) -> (element=w253:u32)
            n128 = Index Array(array=w250, index=w249) -> (element=w248:T24)
            n129 = Unbundle(w248) -> ("Operation"=w247:enum16{"Update", "Clear"})  [unwired: 1 out]
            n130 = local read "Command Selection"() -> (w246:i32)
            n131 = property on="Command Selection" class="MCListbox (strict)"("ActiveCell"=w254, "CellBG"=w253, "ActiveCell"=w252, "CellBG"=w251) -> ()  [unwired: 2 in, 2 out]
            n132 = call <vilib>:"WPI_DashboardUpdate RPC Info.vi"("Operation"=w247) -> ("update"=w245:bool, "commands"=w244:string[][])  [unwired: 9 in]
            n133 = property on="Command Selection" class="MCListbox (strict)"("ItemNames"=w244) -> ()  [unwired: 2 in, 2 out]
            n134 = property on="Command Params" class="Tbl (strict)"("Active Cell"=w254, "Cell BG Color"=w253, "Active Cell"=w252, "Cell BG Color"=w251) -> ()  [unwired: 2 in, 2 out]
            n135 = call <vilib>:"WPI_DashboardUpdate Command Params.vi"("Update"=w245, "NewVal"=w246, "Commands"=w244, "Param Tbl"=w243) -> ()  [unwired: 7 in, 1 out]
          }
        }
        n136 = call <vilib>:"Connextion Info.vi"() -> ("Connected"=→"NT Connection":bool)  [unwired: 10 in, 1 out]
      }
      event "Test Tree": Value Change {
        # "Show appropriate\ncontrols"
        n137 = event-data() -> ("CtlRef"=w260:refnum<vi>, "NewVal"=w258:string)  [unwired: 1 in]
        n138 = call <vilib>:"WPI_UtilitiesGetTreeIOName.vi"("NewVal"=w258, "TreeControl in"=w260) -> ("I/O Name"=w261:string)  [unwired: 9 in]
        n139 = case shown="\"Camera\"" w261 {
          selector: w261 -> [_ w268 _ w290 w299 _]
          tunnel: w258 -> [_ _ w287 w289 _ w306]
          tunnel: cluster{string[]}[] [{["640x480", "320x240", "160x120"]}, {["Auto", "Fixed indoor", "Fixed outdoor 1", "Fixed outdoor 2", "Fixed fluorescent 1", "Fixed fluorescent 2", "Hold current"]}, {["Auto", "Flicker-free 50 Hz", "Flicker-free 60 Hz", "Hold current"]}, {["None", "Prioritize frame rate", "Prioritize image quality"]}, {["Monochrome", "Color"]}] -> [_ _ _ _ _ w305]
          frame Default {
            w263 = FALSE ("Visible")
            w262 = FALSE ("Visible")
            n140 = property on="Motor" class="Clust (strict)"("Visible"=w262) -> ()  [unwired: 2 in, 2 out]
            n141 = property on="Test Ring" class="Ring (strict)"("Visible"=w262) -> ()  [unwired: 2 in, 2 out]
            n142 = property on="Rev/Fwd" class="Clust (strict)"("Visible"=w263) -> ()  [unwired: 2 in, 2 out]
            n143 = property on="On/Off" class="Bool (strict)"("Visible"=w263) -> ()  [unwired: 2 in, 2 out]
            n144 = property on="Test Slider" class="Slide (strict)"("Visible"=w263) -> ()  [unwired: 2 in, 2 out]
          }
          frame "Analog Out", "Motor", "PWM" {
            w269 = FALSE ("Visible")
            n145 = case shown="\"Analog Out\"" w268 {
              tunnel: [1.0 ("Value") -1.0 ("Value") 0.0 ("Value")] -> w267
              tunnel: [255.0 ("Value") 1.0 ("Value") 5.0 ("Value")] -> w266
              tunnel: [128.0 ("Value") 0.0 ("Value") 0.0 ("Value")] -> w265
              tunnel: [64.0 ("Value") 0.5 ("Value") 1.0 ("Value")] -> w264
              frame "PWM" {
              }
              frame "Motor", Default {
              }
              frame "Analog Out" {
              }
            }
            n146 = property on="Motor" class="Clust (strict)"("Visible"=TRUE) -> ()  [unwired: 2 in, 2 out]
            n147 = property on="Value" class="Slide (strict)"("Value"=w265, "Scale.Minimum"=w267, "Scale.Maximum"=w266, "Scale.Increment"=w264) -> ()  [unwired: 2 in, 2 out]
            n148 = property on="On/Off" class="Bool (strict)"("Visible"=w269) -> ()  [unwired: 2 in, 2 out]
            n149 = property on="Test Slider" class="Slide (strict)"("Visible"=w269) -> ()  [unwired: 2 in, 2 out]
            n150 = property on="Test Ring" class="Ring (strict)"("Visible"=w269) -> ()  [unwired: 2 in, 2 out]
            n151 = property on="Rev/Fwd" class="Clust (strict)"("Visible"=w269) -> ()  [unwired: 2 in, 2 out]
          }
          frame "Servo" {
            w285 = FALSE ("Visible")
            n152 = call <vilib>:"NT Read Number.vi"("Name"=w287) -> ("Numeric"=w286:dbl)  [unwired: 9 in, 1 out]
            n153 = property on="Test Slider" class="Slide (strict)"("Visible"=TRUE, "Scale.Maximum"=170.0 ("Scale.Range:Maximum")) -> ()  [unwired: 2 in, 2 out]
            n154 = local write "Test Slider"(w286) -> ()
            n155 = property on="Motor" class="Clust (strict)"("Visible"=w285) -> ()  [unwired: 2 in, 2 out]
            n156 = property on="Rev/Fwd" class="Clust (strict)"("Visible"=w285) -> ()  [unwired: 2 in, 2 out]
            n157 = property on="On/Off" class="Bool (strict)"("Visible"=w285) -> ()  [unwired: 2 in, 2 out]
            n158 = property on="Test Ring" class="Ring (strict)"("Visible"=w285) -> ()  [unwired: 2 in, 2 out]
          }
          frame "Relay", "Solenoid" {
            w288 = FALSE ("Visible")
            n159 = property on="Motor" class="Clust (strict)"("Visible"=w288) -> ()  [unwired: 2 in, 2 out]
            n160 = property on="Test Slider" class="Slide (strict)"("Visible"=w288) -> ()  [unwired: 2 in, 2 out]
            n161 = Search and Replace String(input string=w289, search string="/Value  **", replace string="/Direction") -> (result string=w295:string)  [unwired: 5 in, 3 out]
            n162 = property on="Test Ring" class="Ring (strict)"("Visible"=w288) -> ()  [unwired: 2 in, 2 out]
            n163 = call <vilib>:"NT Read String.vi"("Name"=w295) -> ("String"=w293:string)  [unwired: 9 in, 1 out]
            n164 = Equal?(x="Both directions", y=w293) -> (x = y?=w291:bool)
            n165 = Not(x=w291) -> (.not. x?=w292:bool)
            n166 = property on="Rev/Fwd" class="Clust (strict)"("Visible"=w291) -> ()  [unwired: 2 in, 2 out]
            n167 = property on="On/Off" class="Bool (strict)"("Visible"=w292, "Caption.Text"=w290) -> ()  [unwired: 2 in, 2 out]
          }
          frame "Compressor", "Digital Out" {
            w298 = FALSE ("Visible")
            # "Get direction and finish"
            n168 = property on="Motor" class="Clust (strict)"("Visible"=w298) -> ()  [unwired: 2 in, 2 out]
            n169 = property on="Test Slider" class="Slide (strict)"("Visible"=w298) -> ()  [unwired: 2 in, 2 out]
            n170 = property on="Test Ring" class="Ring (strict)"("Visible"=w298) -> ()  [unwired: 2 in, 2 out]
            n171 = property on="On/Off" class="Bool (strict)"("Visible"=TRUE, "Caption.Text"=w299) -> ()  [unwired: 2 in, 2 out]
            n172 = property on="Rev/Fwd" class="Clust (strict)"("Visible"=FALSE) -> ()  [unwired: 2 in, 2 out]
          }
          frame "Camera" {
            n173 = call <vilib>:"Get Last Path Segment.vi"("String in"=w306) -> ("String out"=w307:string)  [unwired: 10 in]
            n174 = property on="On/Off" class="Bool (strict)"("Visible"=FALSE) -> ()  [unwired: 2 in, 2 out]
            n175 = property on="Motor" class="Clust (strict)"("Visible"=FALSE) -> ()  [unwired: 2 in, 2 out]
            n176 = property on="Rev/Fwd" class="Clust (strict)"("Visible"=FALSE) -> ()  [unwired: 2 in, 2 out]
            n177 = case shown="\"White Balance  **\"" w307 {
              tunnel: w306 -> [w313 w322 w331 w340 w349 _ w355]
              tunnel: w305 -> [w311 w319 w328 w337 w346 _ _]
              frame "Size  **" {
                n178 = Index Array(array=w311) -> (element=w310:cluster{string[]})  [unwired: 1 in]
                n179 = call <vilib>:"NT Read String.vi"("Name"=w313) -> ("String"=w312:string)  [unwired: 9 in, 1 out]
                n180 = Unbundle(w310) -> (w308:string[])
                n181 = Match First String(2:w308, 3:w312) -> (0:w309:i32)  [unwired: 1 out]
                n182 = property on="Test Ring" class="Ring (strict)"("Value"=w309, "Strings []"=w308) -> ()  [unwired: 2 in, 2 out]
                n183 = property on="Test Ring" class="Ring (strict)"("Visible"=TRUE) -> ()  [unwired: 2 in, 2 out]
                n184 = property on="Test Slider" class="Slide (strict)"("Visible"=FALSE) -> ()  [unwired: 2 in, 2 out]
              }
              frame "White Balance  **" {
                n185 = Index Array(array=w319, index=1) -> (element=w320:cluster{string[]})
                n186 = call <vilib>:"NT Read String.vi"("Name"=w322) -> ("String"=w321:string)  [unwired: 9 in, 1 out]
                n187 = Unbundle(w320) -> (w317:string[])
                n188 = Match First String(2:w317, 3:w321) -> (0:w316:i32)  [unwired: 1 out]
                n189 = property on="Test Ring" class="Ring (strict)"("Value"=w316, "Strings []"=w317) -> ()  [unwired: 2 in, 2 out]
                n190 = property on="Test Ring" class="Ring (strict)"("Visible"=TRUE) -> ()  [unwired: 2 in, 2 out]
                n191 = property on="Test Slider" class="Slide (strict)"("Visible"=FALSE) -> ()  [unwired: 2 in, 2 out]
              }
              frame "Exposure  **" {
                n192 = Index Array(array=w328, index=2) -> (element=w329:cluster{string[]})
                n193 = call <vilib>:"NT Read String.vi"("Name"=w331) -> ("String"=w330:string)  [unwired: 9 in, 1 out]
                n194 = Unbundle(w329) -> (w325:string[])
                n195 = Match First String(2:w325, 3:w330) -> (0:w326:i32)  [unwired: 1 out]
                n196 = property on="Test Ring" class="Ring (strict)"("Value"=w326, "Strings []"=w325) -> ()  [unwired: 2 in, 2 out]
                n197 = property on="Test Ring" class="Ring (strict)"("Visible"=TRUE) -> ()  [unwired: 2 in, 2 out]
                n198 = property on="Test Slider" class="Slide (strict)"("Visible"=FALSE) -> ()  [unwired: 2 in, 2 out]
              }
              frame "Exposure Priority  **" {
                n199 = Index Array(array=w337, index=3) -> (element=w338:cluster{string[]})
                n200 = call <vilib>:"NT Read String.vi"("Name"=w340) -> ("String"=w339:string)  [unwired: 9 in, 1 out]
                n201 = Unbundle(w338) -> (w334:string[])
                n202 = Match First String(2:w334, 3:w339) -> (0:w335:i32)  [unwired: 1 out]
                n203 = property on="Test Ring" class="Ring (strict)"("Value"=w335, "Strings []"=w334) -> ()  [unwired: 2 in, 2 out]
                n204 = property on="Test Ring" class="Ring (strict)"("Visible"=TRUE) -> ()  [unwired: 2 in, 2 out]
                n205 = property on="Test Slider" class="Slide (strict)"("Visible"=FALSE) -> ()  [unwired: 2 in, 2 out]
              }
              frame "Color Enable  **" {
                n206 = Index Array(array=w346, index=4) -> (element=w347:cluster{string[]})
                n207 = call <vilib>:"NT Read String.vi"("Name"=w349) -> ("String"=w348:string)  [unwired: 9 in, 1 out]
                n208 = Unbundle(w347) -> (w343:string[])
                n209 = Match First String(2:w343, 3:w348) -> (0:w344:i32)  [unwired: 1 out]
                n210 = property on="Test Ring" class="Ring (strict)"("Value"=w344, "Strings []"=w343) -> ()  [unwired: 2 in, 2 out]
                n211 = property on="Test Ring" class="Ring (strict)"("Visible"=TRUE) -> ()  [unwired: 2 in, 2 out]
                n212 = property on="Test Slider" class="Slide (strict)"("Visible"=FALSE) -> ()  [unwired: 2 in, 2 out]
              }
              frame Default {
                n213 = property on="Test Ring" class="Ring (strict)"("Visible"=FALSE) -> ()  [unwired: 2 in, 2 out]
                n214 = property on="Test Slider" class="Slide (strict)"("Visible"=FALSE) -> ()  [unwired: 2 in, 2 out]
              }
              frame "Brightness  **", "Color Level  **", "Compression  **", "FPS  **", "Sharpness  **" {
                n215 = call <vilib>:"NT Read Number.vi"("Name"=w355) -> ("Numeric"=w354:dbl)  [unwired: 9 in, 1 out]
                n216 = local write "Test Slider"(w354) -> ()
                n217 = property on="Test Slider" class="Slide (strict)"("Visible"=TRUE, "Scale.Maximum"=100.0 ("Scale.Range:Maximum")) -> ()  [unwired: 2 in, 2 out]
                n218 = property on="Test Ring" class="Ring (strict)"("Visible"=FALSE) -> ()  [unwired: 2 in, 2 out]
              }
            }
          }
        }
        n219 = property on="Progress" class="Clust (strict)"("Visible"=FALSE) -> ()  [unwired: 2 in, 2 out]
      }
      event "Test Name": Mouse Enter {
        # "Populate the ring with the list of tests"
        n220 = event-data() -> ()  [unwired: 1 in, 1 out]
        n221 = call <vilib>:"NT Read String Array.vi"("Name"="TestMode/TestList") -> ("String Array"=w363:string[])  [unwired: 9 in, 1 out]
        n222 = Build Array (concatenate)("Select the test to run...", w363) -> (w362:string[])
        n223 = property on="Test Name" class="Ring (strict)"("Strings []"=w362) -> ()  [unwired: 2 in, 2 out]
      }
      event "Test Name": Value Change {
        w365 = FALSE ("Visible")
        # "Tell the robot the test name to run"
        n224 = event-data() -> ("NewVal"=w369:u16)  [unwired: 1 in]
        n225 = property on="Test Name" class="Ring (strict)"() -> ("Strings []"=w370:string[])  [unwired: 2 in, 2 out]
        n226 = local write "Progress"(T6 {"Test Progress"=0, "Test Progress Text"=""} ("Progress")) -> ()
        n227 = Index Array(array=w370, index=w369) -> (element=w368:string)
        n228 = call <vilib>:"NT Write String.vi"("String"=w368, "Name"="TestMode/TestName") -> ()  [unwired: 9 in, 1 out]
        n229 = property on="Progress" class="Clust (strict)"("Visible"=TRUE) -> ()  [unwired: 2 in, 2 out]
        n230 = property on="Motor" class="Clust (strict)"("Visible"=w365) -> ()  [unwired: 2 in, 2 out]
        n231 = property on="Test Slider" class="Slide (strict)"("Visible"=w365) -> ()  [unwired: 2 in, 2 out]
        n232 = property on="On/Off" class="Bool (strict)"("Visible"=w365) -> ()  [unwired: 2 in, 2 out]
        n233 = property on="Rev/Fwd" class="Clust (strict)"("Visible"=w365) -> ()  [unwired: 2 in, 2 out]
        n234 = property on="Test Ring" class="Ring (strict)"("Visible"=w365) -> ()  [unwired: 2 in, 2 out]
      }
      event "Select Auto": Mouse Enter {
        # "Populate the combo box with the list of autonomous options"
        n235 = event-data() -> ()  [unwired: 1 in, 1 out]
        n236 = call <vilib>:"NT Read String Array.vi"("Name"="Auto List") -> ("String Array"=w372:string[])  [unwired: 9 in, 1 out]
        n237 = property on="Select Auto" class="CmbBox"("Strings[]"=w372) -> ()  [unwired: 2 in, 2 out]
      }
      event "Select Auto": Value Change {
        # "User modified the Auto Selection. Write to NT variable so robot knows."
        n238 = event-data() -> ("NewVal"=w375:string)  [unwired: 1 in]
        n239 = call <vilib>:"NT Write String.vi"("String"=w375, "Name"="Auto Selector") -> ()  [unwired: 9 in, 1 out]
      }
      event "Command Selection": Value Change {
        # "Get the params and show in table"
        n240 = event-data() -> ("NewVal"=w381:i32)  [unwired: 1 in]
        n241 = property on="Command Selection" class="MCListbox (strict)"() -> ("ItemNames"=w379:string[][])  [unwired: 2 in, 2 out]
        n242 = call <vilib>:"WPI_DashboardUpdate Command Params.vi"("NewVal"=w381, "Commands"=w379, "Param Tbl"=w380) -> ()  [unwired: 8 in, 1 out]
      }
      event "Execute Command": Value Change {
        # "Started one, Unique ID holds\nresponse"
        n243 = event-data() -> ()  [unwired: 1 in, 1 out]
        n244 = property on="Command Selection" class="MCListbox (strict)"() -> ("ItemNames"=w392:string[][])  [unwired: 2 in, 2 out]
        n245 = Index Array(array=w392, index (row)="Command Selection", index (col)=0) -> (element=w390:string)
        n246 = call <vilib>:"Invoke Commands.vi"("Command Params"="Command Params", "Function Name"=w390) -> ("Params"=w386:u8, "Started"=w385:bool)  [unwired: 7 in, 1 out]
        n247 = Array Subset(array="Command Params", length (row)=w386) -> (w387:string[][])  [unwired: 3 in]
        n248 = Select(t="Executing" ("Cmd Status"), s=w385, f="" ("Cmd Status")) -> (s? t:f=→"Cmd Status":string)
      }
      event "Command Selection": Double Click {
        n249 = event-data() -> ("Row"=w400:i32)  [unwired: 1 in]
        n250 = property on="Command Selection" class="MCListbox (strict)"() -> ("ItemNames"=w403:string[][])  [unwired: 2 in, 2 out]
        n251 = local read "Command Params"() -> (w399:string[][])
        n252 = Index Array(array=w403, index (row)=w400, index (col)=0) -> (element=w401:string)
        n253 = call <vilib>:"Invoke Commands.vi"("Command Params"=w399, "Function Name"=w401) -> ("Params"=w398:u8, "Started"=w393:bool)  [unwired: 7 in, 1 out]
        n254 = Array Subset(array=w399, length (row)=w398) -> (w397:string[][])  [unwired: 3 in]
        n255 = Select(t="Executing" ("Cmd Status"), s=w393, f="" ("Cmd Status")) -> (s? t:f=w394:string)
        n256 = local write "Cmd Status"(w394) -> ()
      }
      event "CheckList": Double Click {
        # "Shift clears all"
        # "Update symbols on the listbox"
        n257 = event-data() -> ("PlatMods.Shift"=w405:bool, "Row"=w407:i32)  [unwired: 1 in]
        n258 = case shown="True" w405 {
          tunnel: w407 -> [w411 _]
          tunnel: 1 -> [w410 _]
          frame False {
            n259 = property on="CheckList" class="LstBox (strict)"() -> ("Item Symbols"=w409:i32[])  [unwired: 2 in, 2 out]
            n260 = Replace Array Subset(array=w409, new element=w410, index=w411) -> (w408:i32[])
            n261 = property on="CheckList" class="LstBox (strict)"("Item Symbols"=w408) -> ()  [unwired: 2 in, 2 out]
          }
          frame True {
            w412 = 0 ("Top Row")
            n262 = property on="CheckList" class="LstBox (strict)"() -> ("Number of Rows"=w414:u32)  [unwired: 2 in, 2 out]
            n263 = Initialize Array(0, w414) -> (w413:i32[])
            n264 = property on="CheckList" class="LstBox (strict)"("Top Row"=w412, "Value"=w412, "Item Symbols"=w413) -> ()  [unwired: 2 in, 2 out]
          }
        }
      }
      event "CheckList": Key Down {
        # "Update symbols on the listbox\nLeft and right keys check and uncheck"
        n265 = event-data() -> ("VKey"=w418:T22)  [unwired: 1 in]
        n266 = case shown="\"Left\", \"Right\"" w418 {
          selector: w418 -> [w423 _]
          tunnel: eventvkey."Left" ("VKey") -> [w421 _]
          frame "Left", "Right" {
            n267 = Equal?(x=w421, y=w423) -> (x = y?=w422:bool)
            n268 = Select(t=0, s=w422, f=1) -> (s? t:f=w424:i32)
            n269 = property on="CheckList" class="LstBox (strict)"() -> ("Item Symbols"=w427:i32[])  [unwired: 2 in, 2 out]
            n270 = Replace Array Subset(array=w427, new element=w424, index="CheckList") -> (w426:i32[])
            n271 = property on="CheckList" class="LstBox (strict)"("Item Symbols"=w426) -> ()  [unwired: 2 in, 2 out]
          }
          frame Default {
          }
        }
      }
      event "Motor.Enable": Value Change {
        # "When the test mode otor enable helper is set, update that\ntree row item's value"
        n272 = event-data() -> ("NewVal"=w433:bool)  [unwired: 1 in]
        n273 = Unbundle("Motor") -> ("Value"=w432:dbl)  [unwired: 1 out]
        n274 = Select(t=w432, s=w433, f=0.0) -> (s? t:f=w430:dbl)
        n275 = call <vilib>:"NT Write Number.vi"("Numeric"=w430, "Name"=w429) -> ()  [unwired: 9 in, 1 out]
      }
      event "Test Slider": Value Change {
        # "When the test mode slider helper is set, update that\ntree row item's value"
        n276 = event-data() -> ("NewVal"=w436:dbl)  [unwired: 1 in]
        n277 = call <vilib>:"NT Write Number.vi"("Numeric"=w436, "Name"=w437) -> ()  [unwired: 9 in, 1 out]
      }
      event "On/Off": Value Change {
        # "When the test mode on/off helper value is set, update that\ntree row item's value"
        n278 = event-data() -> ("NewVal"=w441:bool)  [unwired: 1 in]
        n279 = Boolean To (0,1)(Boolean=w441) -> (0, 1=w440:i16)
        n280 = call <vilib>:"NT Write Number.vi"("Numeric"=w440, "Name"=w439) -> ()  [unwired: 9 in, 1 out]
      }
      event "Rev/Fwd": Value Change {
        # "When the test mode helper value for relays is set, update that\ntree row item's value"
        n281 = event-data() -> ("NewVal.Forward"=w449:bool, "NewVal.Reverse"=w448:bool)  [unwired: 1 in]
        n282 = Boolean To (0,1)(Boolean=w449) -> (0, 1=w445:i16)
        n283 = Boolean To (0,1)(Boolean=w448) -> (0, 1=w447:i16)
        n284 = Negate(x=w447) -> (-x=w446:i16)
        n285 = Add(x=w445, y=w446) -> (x+y=w444:i16)
        n286 = call <vilib>:"NT Write Number.vi"("Numeric"=w444, "Name"=w443) -> ()  [unwired: 9 in, 1 out]
      }
      event "Test Ring": Value Change {
        # "When a test mode helper value is selected from the ring,\nset the tree item's variable to the string value"
        n287 = event-data() -> ("NewVal"=w453:u16)  [unwired: 1 in]
        n288 = property on="Test Ring" class="Ring (strict)"() -> ("Strings []"=w454:string[])  [unwired: 2 in, 2 out]
        n289 = Index Array(array=w454, index=w453) -> (element=w452:string)
        n290 = call <vilib>:"NT Write String.vi"("String"=w452, "Name"=w451) -> ()  [unwired: 9 in, 1 out]
      }
      event "Rec Mode": Value Change {
        # "Update globals for recording mode and path to read log from.\nClear when logging and let NetworkTables set path for vision to\nuse."
        n291 = event-data() -> ("NewVal"=w465:enum32{"Stop", "Record", "Playback"})  [unwired: 1 in]
        n292 = global write "WPI_DashboardLogging Global.vi" "Logging Filename"(path "") -> ()
        n293 = global write "WPI_DashboardLogging Global.vi" "Recording"(w465) -> ()
        n294 = case shown="\"Playback\"" w465 {
          tunnel: w464 -> [_ w467 w476]
          tunnel: [_ _ w475] -> w462
          tunnel: [_ _ w474] -> _
          tunnel: w460 -> [_ _ w472]
          tunnel: cluster{i32, i32} {-250, 170} -> [_ _ w471]
          tunnel: [_ _ T23 {"Image Size"=TRUE, "Image Type"=TRUE, "Pixel Value"=TRUE, "ROI Information"=TRUE, "Zoom Factor"=FALSE} ("Image Information Shown:All Elements")] -> w455
          tunnel: [_ _ TRUE ("Zoom Factor")] -> w456
          tunnel: w458 -> [_ _ w468]
          frame Default {
          }
          frame "Stop", "Record" {
            # "Place Window too"
            n295 = invoke class="VI" method="FP.Close"(reference=w467) -> (reference out=w466:refnum<vi>)  [unwired: 2 in, 2 out]
            n296 = invoke class="VI" method="Abort VI"(reference=w466) -> ()  [unwired: 2 in, 3 out]
          }
          frame "Playback" {
            n297 = call "Open Playback Panel.vi"("Offset"=w471, "DB VI Ref"=w472, "Playback in"=w476) -> ("Playback out"=w473:refnum<vi>)  [unwired: 8 in]
            n298 = register-events(w473, w468) -> (reference out=w475:refnum<event-registration>, error out=w474:errorcluster)  [unwired: 2 in]
          }
        }
        n299 = property on="Camera Image Right" class="ImageControl"("Image Information Shown"=w455, "Image Information Visible"=w456) -> ()  [unwired: 2 in, 2 out]
        n300 = property on="Camera Image" class="ImageControl"("Image Information Shown"=w455, "Image Information Visible"=w456) -> ()  [unwired: 2 in, 2 out]
        n301 = call <vilib>:"WPI_DashboardNT Log FieldName Cache.vi"("Operation"=enum16{"Lookup/Add", "Index", "Clear"}."Clear") -> ()  [unwired: 8 in, 3 out]
      }
      event Panel Close {
        w478 = enum32{"Stop", "Record", "Playback"}."Stop" ("Rec Mode")
        # "Playback window has been closed, abort"
        n302 = event-data() -> ()  [unwired: 1 in, 4 out]
        n303 = local write "Rec Mode"(w478) -> ()
        n304 = global write "WPI_DashboardLogging Global.vi" "Recording"(w478) -> ()
      }
      event Panel Close {
        # "Abort playback window and ourself"
        n305 = event-data() -> ()  [unwired: 1 in, 4 out]
        n306 = invoke class="VI" method="FP.Close"(reference=w482) -> (reference out=w481:refnum<vi>)  [unwired: 2 in, 2 out]
        n307 = invoke class="VI" method="Abort VI"(reference=w481) -> (error out=w480:errorcluster)  [unwired: 2 in, 2 out]
        n308 = invoke class="VI" method="Abort VI"(error in=w480) -> ()  [unwired: 2 in, 3 out]
      }
      event User Event {
        n309 = event-data() -> ("IDs"=w489:cluster{"RPC field ID":u16, "Unique ID":u16}, "String"=w488:string)  [unwired: 1 in]
        n310 = Bundle("IDs"=w489, "String"=w488) -> (w487:T9)  [unwired: 1 in]
        n311 = call <vilib>:"Retrieve RPC Response.vi"("RPC Response"=w487) -> ("Output"=w485:string[][])  [unwired: 10 in]
        n312 = Build Array (concatenate)(w483, w485) -> (w484:string[][])
        n313 = local write "Command Params"(w484) -> ()
        n314 = local write "Cmd Status"("" ("Cmd Status")) -> ()
      }
      event "Tree": Double Click {
        n315 = event-data() -> ("PlatMods"=w495:T26, "Tag"=w492:string)  [unwired: 1 in]
        n316 = Unbundle(w495) -> ("Shift"=w494:bool)  [unwired: 4 out]
        n317 = String Subset(string=w492, length (rest)=1 ("length (rest)")) -> (substring=w491:string)  [unwired: 1 in]
        n318 = Not(x=w494) -> (.not. x?=w493:bool)
        n319 = case shown="\"/\"" w491 {
          tunnel: w492 -> [_ w498]
          tunnel: w493 -> [_ w497]
          frame Default {
          }
          frame "/" {
            n320 = call <vilib>:"NT Update Persistence.vi"("Persistence"=w497, "Name"=w498) -> ()  [unwired: 9 in, 1 out]
          }
        }
      }
    }
  }
  n321 = while {
    tunnel: w65 -> [w500]
    i -> [w503]
    stop <- FALSE stop-if-true
    n322 = Wait (ms)(milliseconds to wait=u32 100) -> ()  [unwired: 1 out]
    n323 = case shown="\"Playback\"" "Rec Mode" {
      tunnel: w503 -> [_ _ w518]
      tunnel: [u32 2829099 ("Base Color") u32 11141120 ("Target Color") w507] -> w499
      frame "Stop", Default {
        # "Reset the color, extra updates don't cost much"
      }
      frame "Record" {
      }
      frame "Playback" {
        # "Playback"
        n324 = Quotient & Remainder(x=w518, y=u32 50 ("milliseconds to wait")) -> (x-y*floor(x/y)=w514:u32)  [unwired: 1 out]
        n325 = Divide(x=w514, y=u32 50 ("milliseconds to wait")) -> (x/y=w511:dbl)
        n326 = Multiply(x=6.283185307179586, y=w511) -> (x*y=w516:dbl)
        n327 = Sine(x=w516) -> (sin(x)=w515:dbl)
        n328 = Absolute Value(x=w515) -> (abs(x)=w508:dbl)
        n329 = call "Interpolate RGB Color.vi"("Proportion"=w508, "Target Color"=u32 30976, "Base Color"=u32 2829099) -> ("Result Color"=w507:u32)  [unwired: 8 in]
      }
    }
    n330 = property class="Pane"(reference=w500, "PaneColor"=w499) -> ()  [unwired: 1 in, 2 out]
  }
  n331 = local write "Dashboard Tab"(T2."Drive" ("Dashboard Tab")) -> ()
  n332 = property on="On/Off" class="Bool (strict)"("Visible"=w36) -> ()  [unwired: 2 in, 2 out]
  n333 = property on="Motor" class="Clust (strict)"("Visible"=w36) -> ()  [unwired: 2 in, 2 out]
  n334 = property on="Progress" class="Clust (strict)"("Visible"=w36) -> ()  [unwired: 2 in, 2 out]
  n335 = property on="Test Ring" class="Ring (strict)"("Visible"=w36) -> ()  [unwired: 2 in, 2 out]
  n336 = property on="Rev/Fwd" class="Clust (strict)"("Visible"=w36) -> ()  [unwired: 2 in, 2 out]
  n337 = while {
    tunnel: u16 1741 ("timeout ms (25000)") -> [w520]
    stop <- FALSE stop-if-true
    n338 = TCP Create Listener(10:w520) -> (0:w519:errorcluster, 3:w521:refnum<k5>)  [unwired: 4 in, 1 out]
    n339 = case shown="No Error" w519 {
      selector: w519 -> [w523 _]
      tunnel: w521 -> [w524 _]
      frame No Error {
        n340 = while {
          tunnel: w524 -> [w527]
          tunnel: w523 -> [w526]
          stop <- FALSE stop-if-true
          n341 = TCP Wait On Listener(8:w526, 11:w527) -> (0:w528:errorcluster, 4:w529:refnum<k5>)  [unwired: 2 in, 3 out]
          n342 = local write "TCP"(w529) -> ()
          n343 = case shown="No Error" w528 {
            frame No Error {
            }
            frame Error {
              n344 = Wait (ms)(milliseconds to wait=u32 1000) -> ()  [unwired: 1 out]
            }
          }
        }
      }
      frame Error {
        n345 = Wait (ms)(milliseconds to wait=u32 1000) -> ()  [unwired: 1 out]
      }
    }
  }
  n346 = local write "Command Selection"(u16 0 ("milliseconds to wait")) -> ()
  n347 = local write "Command Params"(string[][] [] ("Command Params")) -> ()
  n348 = global write "WPI_DashboardLogging Global.vi" "Recording"(w59) -> ()
  n349 = local write "Rec Mode"(w59) -> ()
  n350 = call <vilib>:"NT Write String.vi"("String"="Select Auto", "Name"="Auto Selector") -> ()  [unwired: 9 in, 1 out]
